vi "Launch.vi"(8 "error in (no error)":errorcluster, 10 "Run":bool, 11 "Source Instr in":refnum<class "Source Instr.lvclass">) -> (0 "error out":errorcluster, 3 "Source Instr out":refnum<class "Source Instr.lvclass">)   [LabVIEW 2015, in "Item Actor.lvlib" / "Source Instr.lvclass"]
uses:
  Source Instr.lvclass
  Instrument Information/Instrument.lvclass/Instrument.ctl
  <userlib>/_SmartBalloon/Balloon Generic/Aesthetics.ctl
  Instrument Information/Read App Path.vi
  <userlib>/_SmartBalloon/Symbol Text Balloon/Symbol Text Balloon.lvclass
  <userlib>/_SmartBalloon/Balloon Generic/Balloon.lvclass
  <userlib>/_SmartBalloon/Engine/Engine.lvclass
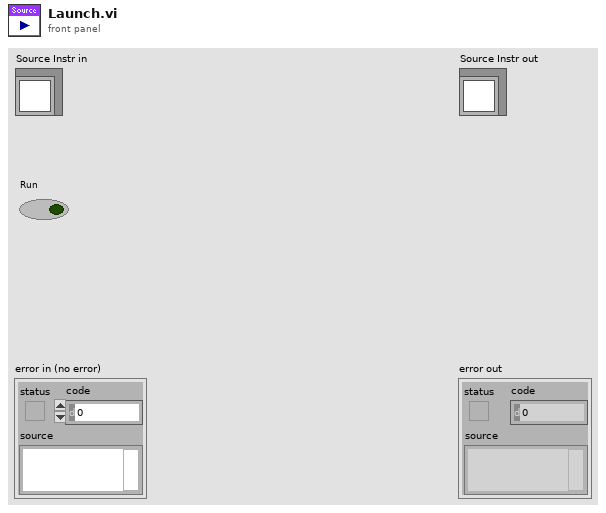
[diagram p1: front panel]
types:
  T1 = typedef "Balloon Engine.lvlib/Balloon.lvclass/Aesthetics.ctl" = cluster{"Colors":cluster{"Font Color":u32, "Panel Color":u32}, "Position":enum16{"Top", "Bottom"}, "Display Time (ms)":i32}
  T2 = enum32{"Bad", "Idle", "Run top level", "Running"}
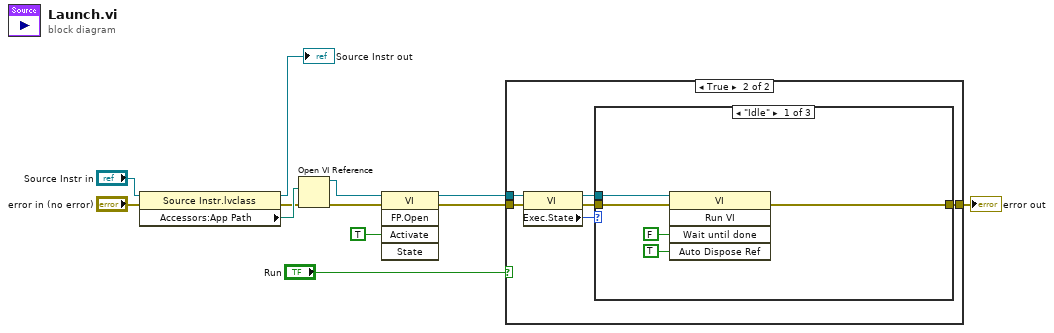
[diagram p0: block diagram]
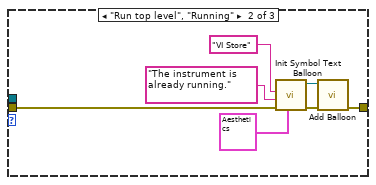
[diagram p3: hidden frame]
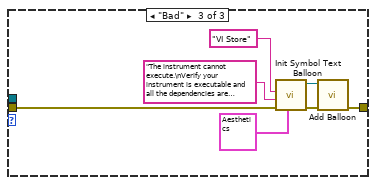
[diagram p4: hidden frame]
diagram:
  n1 = property class="Source Instr.lvclass"(reference="Source Instr in", error in="error in (no error)") -> (reference out=→"Source Instr out":refnum<class "Source Instr.lvclass">, error out=w9:errorcluster, "Accessors:App Path"=w10:path)
  n2 = Open VI Reference(vi path=w10, error in (no error)=w9) -> (vi reference=w5:refnum<vi>, error out=w1:errorcluster)  [unwired: 4 in]
  n3 = invoke class="VI" method="FP.Open"(reference=w5, error in=w1, "Activate"=TRUE ("Activate?")) -> (reference out=w3:refnum<vi>, error out=w2:errorcluster)  [unwired: 2 in, 3 out]
  n4 = case shown="True" "Run" {
    tunnel: w2 -> [w13 w19]
    tunnel: w3 -> [_ w18]
    tunnel: [w13 w14] -> w8
    frame False {
    }
    frame True {
      n5 = property class="VI"(reference=w18, error in=w19) -> (reference out=w17:refnum<vi>, error out=w15:errorcluster, "Exec.State"=w16:T2)
      n6 = case shown="\"Idle\"" w16 {
        tunnel: w17 -> [w24 _ _]
        tunnel: w15 -> [w23 w25 w32]
        tunnel: [w20 w26 w34] -> w14
        frame "Idle" {
          n7 = invoke class="VI" method="Run VI"(reference=w24, error in=w23, "Wait until done"=FALSE ("Wait Until Done"), "Auto Dispose Ref"=TRUE ("Auto Dispose Reference")) -> (error out=w20:errorcluster)  [unwired: 1 in, 4 out]
        }
        frame "Run top level", "Running" {
          n8 = call <userlib>:"Init Symbol Text Balloon.vi"("Aesthetics"=T1 {"Colors"={"Font Color"=3305861, "Panel Color"=16246744}, "Position"=enum."Bottom", "Display Time (ms)"=3000}, "error in (no error)"=w25, "Body"="The instrument is already running.", "Title"="VI Store") -> ("error out"=w27:errorcluster, "Symbol Text Balloon out"=w28:refnum<class "Symbol Text Balloon.lvclass">)  [unwired: 6 in]
          n9 = call <userlib>:"Add Balloon.vi"("error in (no error)"=w27, "Next Balloon"=w28) -> ("error out"=w26:errorcluster)  [unwired: 9 in]
        }
        frame "Bad" {
          n10 = call <userlib>:"Init Symbol Text Balloon.vi"("Aesthetics"=T1 {"Colors"={"Font Color"=3305861, "Panel Color"=16246744}, "Position"=enum."Bottom", "Display Time (ms)"=3000}, "error in (no error)"=w32, "Body"="The instrument cannot execute.\nVerify your instrument is executable and all the dependencies are resolved.", "Title"="VI Store") -> ("error out"=w35:errorcluster, "Symbol Text Balloon out"=w36:refnum<class "Symbol Text Balloon.lvclass">)  [unwired: 6 in]
          n11 = call <userlib>:"Add Balloon.vi"("error in (no error)"=w35, "Next Balloon"=w36) -> ("error out"=w34:errorcluster)  [unwired: 9 in]
        }
      }
    }
  }
  "error out" <- w8
